vi "Lock Instrument.vi"(8 "error in (no error)":errorcluster, 9 "Mouse and Touch Screen Lock (F: Unlock)":bool, 10 "Keyboard Lock (F: Unlock)":bool, 11 "VISA resource name":refnum<visa-resource-name>) -> (0 "error out":errorcluster, 3 "VISA resource name out":refnum<visa-resource-name>)   [LabVIEW 2022 SP3, in "Agilent ENA Series.lvlib"]
doc: "Locks or unlocks human interface devices.\n\n<b>Note:</b>\nThis VI is not supported by the E5080A and E5080B."
uses:
  <instrlib>/Agilent ENA Series/Agilent ENA Series.lvlib
panel:
  # "Note:\nThis VI is not supported by E5080A and E5080B."
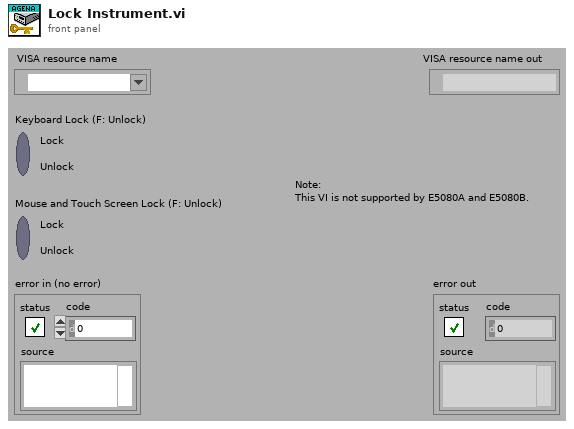
[diagram p1: front panel]
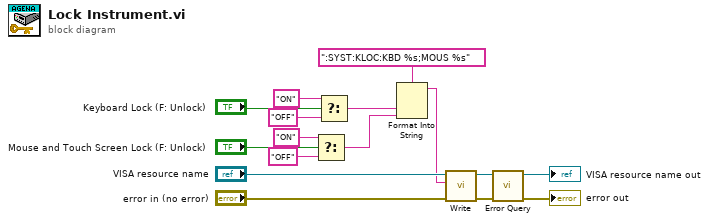
[diagram p0: block diagram]
diagram:
  n1 = Select(t="ON", s="Mouse and Touch Screen Lock (F: Unlock)", f="OFF") -> (s? t:f=w5:string)
  n2 = Select(t="ON", s="Keyboard Lock (F: Unlock)", f="OFF") -> (s? t:f=w6:string)
  n3 = Format Into String(format string=":SYST:KLOC:KBD %s;MOUS %s", w6, w5) -> (resulting string=w13:string)  [unwired: 2 in, 1 out]
  n4 = call <instrlib>:"Write.vi"("error in (no error)"="error in (no error)", "String ()"=w13, "VISA resource name"="VISA resource name") -> ("error out"=w3:errorcluster, "VISA resource name out"=w4:refnum<visa-resource-name>)  [unwired: 6 in, 1 out]
  n5 = call <instrlib>:"Error Query.vi"("error in (no error)"=w3, "VISA resource name"=w4) -> ("error out"=→"error out":errorcluster, "VISA resource name out"=→"VISA resource name out":refnum<visa-resource-name>)  [unwired: 6 in, 2 out]
